vi "Trasnpose_matrix(SubVI).vi"(9 "Line 3":sgl[](array[numeric])=[0.0, 0.0, 0.0], 10 "Line 2":sgl[](array[numeric])=[0.0, 0.0, 0.0], 11 "Line 1":sgl[](array[numeric])=[0.0, 0.0, 0.0]) -> (1 "Line 3 transpose":sgl[](array[numeric]), 2 "Line 2 transpose":sgl[](array[numeric]), 3 "Line 1 transpose":sgl[](array[numeric]))   [LabVIEW 2017]
panel:
  # "Inputs are the lines of a 3x3 matrix"
  # "Outputs are new lines composed by the transpose of the input matrix"
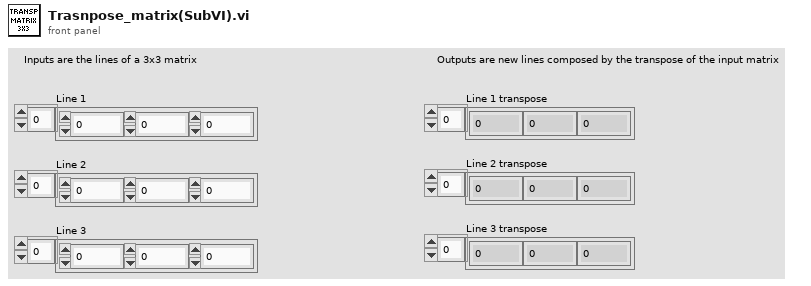
[diagram p1: front panel]
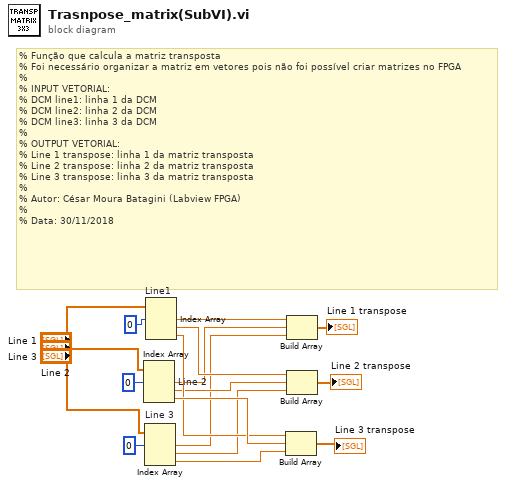
[diagram p0: block diagram]
diagram:
  # "% Função que calcula a matriz transposta\n% Foi necessário organizar a matriz em vetores pois não foi possível criar matrizes no FPGA\n%\n% INPUT VETORIAL: \n% DCM line1: linha 1 da DCM\n% DCM line2: linha 2 da DCM\n% DCM line3: linha 3 da DCM\n%\n% OUTPUT VETORIAL:\n% Line 1 transpose: linha 1 da matriz transposta\n% Line 2 transpose: linha 2 da matriz transposta\n% Line 3 transpose: linha 3 da matriz transposta\n%\n% Autor: César Moura Batagini (Labview FPGA)\n%             \n% Data: 30/11/2018"
  n1 = Index Array "Line 2"(array="Line 2", index #1=0 ("index")) -> (element #1=w8:sgl, element #2=w11:sgl, element #3=w14:sgl)  [unwired: 2 in]
  n2 = Index Array "Line 3"(array="Line 3", index #1=0 ("index")) -> (element #1=w9:sgl, element #2=w12:sgl, element #3=w15:sgl)  [unwired: 2 in]
  n3 = Index Array "Line1"(array="Line 1", index #1=0 ("index")) -> (element #1=w7:sgl, element #2=w10:sgl, element #3=w13:sgl)  [unwired: 2 in]
  n4 = Build Array(w13, w14, w15) -> (→"Line 3 transpose":sgl[])
  n5 = Build Array(w7, w8, w9) -> (→"Line 1 transpose":sgl[])
  n6 = Build Array(w10, w11, w12) -> (→"Line 2 transpose":sgl[])
